vi "Static Error Handling.Source Buffer.Write.Numeric.Base10.Scalar (DBL).vi"(7 "precision (3)":i16=3, 9 "offset":i32, 10 "value":dbl, 11 "error in":errorcluster) -> (1 "new offset":i32, 3 "error out":errorcluster)   [LabVIEW 2016, in "Static Error Handling.lvlib"]
doc: "Converts <b>value</b> into an decimal-formatted string, and writes the string to the <b>error in</b> source buffer at the specified <b>offset</b>."
uses:
  Static Error Handling.lvlib
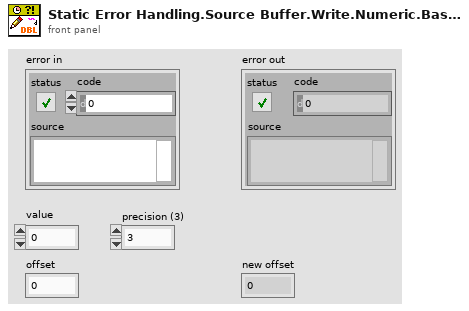
[diagram p1: front panel]
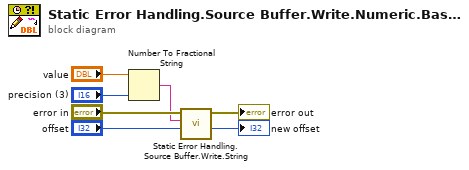
[diagram p0: block diagram]
diagram:
  n1 = Number To Fractional String(number="value", precision (6)="precision (3)") -> (F-format string=w3:string)  [unwired: 2 in]
  n2 = call "Static Error Handling.Source Buffer.Write.String.vi"("offset (0)"="offset", "string"=w3, "error in"="error in") -> ("new offset"=→"new offset":i32, "error out"=→"error out":errorcluster)  [unwired: 7 in]
